vi "counter.vi"() -> ()   [LabVIEW 2023]
panel:
  in  "reset":bool
  out "Counter":i8
  in  "--":bool
  out "Numeric":i32
  in  "stop":bool
  in  "++":bool
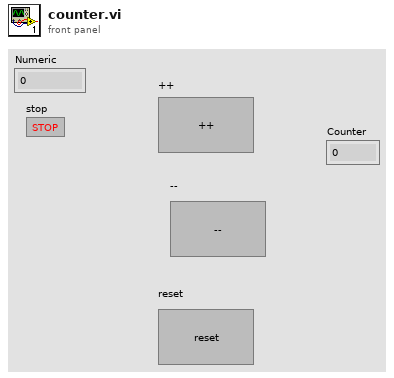
[diagram p1: front panel]
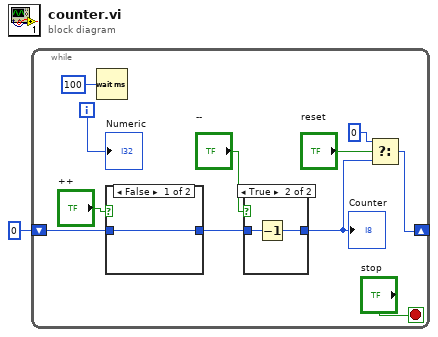
[diagram p0: block diagram]
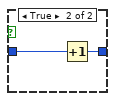
[diagram p3: hidden frame]
diagram:
  n1 = while {
    shift-right: [w4] -> _
    shift-left: i8 0 -> [w8]
    i -> [w11]
    stop <- "stop" stop-if-true
    n2 = Wait (ms)(milliseconds to wait=u32 100) -> ()  [unwired: 1 out]
    n3 = case shown="False" "++" {
      tunnel: w8 -> [w16 w18]
      tunnel: [w16 w17] -> w6
      frame False {
      }
      frame True {
        n4 = Increment(x=w18) -> (x+1=w17:i8)
      }
    }
    n5 = case shown="True" "--" {
      tunnel: w6 -> [w13 w15]
      tunnel: [w13 w14] -> w5
      frame False {
      }
      frame True {
        n6 = Decrement(x=w15) -> (x-1=w14:i8)
      }
    }
    "Counter" <- w5
    n7 = Select(t=i8 0, s="reset", f=w5) -> (s? t:f=w4:i8)
    "Numeric" <- w11
  }
